vi "RES_HPSetup.vi"(8 "error in (no error)":errorcluster, 9 "Data Cluster In":T3 {"GUI Data Cluster"."SBR" format="%08b"}, 10 "Config Cluster In":T1={"General"={"Config.ini"=path "", "Default Logging Path"=path ""}, "Hardware"={"Measure Rate (1/s)"=0, "HP DMM VISA"="", "LS 335 VISA"="", "HP DM"={"Range"=enum."Autorange", "Autozero"=FALSE, "Display"=enum."3 1/2 Digit", "Blank LCD"=FALSE}}, "Operation"={"Operation Mode"=enum."Logging", "Status"="", "NewLog?"=FALSE, "OvenWarn"=FALSE}}) -> (0 "error out":errorcluster, 1 "Data Cluster Out":T3 {"GUI Data Cluster"."SBR" format="%08b"}, 2 "Config Cluster Out":T1={"General"={"Config.ini"=path "", "Default Logging Path"=path ""}, "Hardware"={"Measure Rate (1/s)"=0, "HP DMM VISA"="", "LS 335 VISA"="", "HP DM"={"Range"=enum."Autorange", "Autozero"=FALSE, "Display"=enum."3 1/2 Digit", "Blank LCD"=FALSE}}, "Operation"={"Operation Mode"=enum."Idle-Off", "Status"="", "NewLog?"=FALSE, "OvenWarn"=FALSE}})   [LabVIEW 2021]
uses:
  Config_Cluster.ctl
  Mode_Enum.ctl
  Data_Cluster.ctl
  Measurement_Cluster.ctl
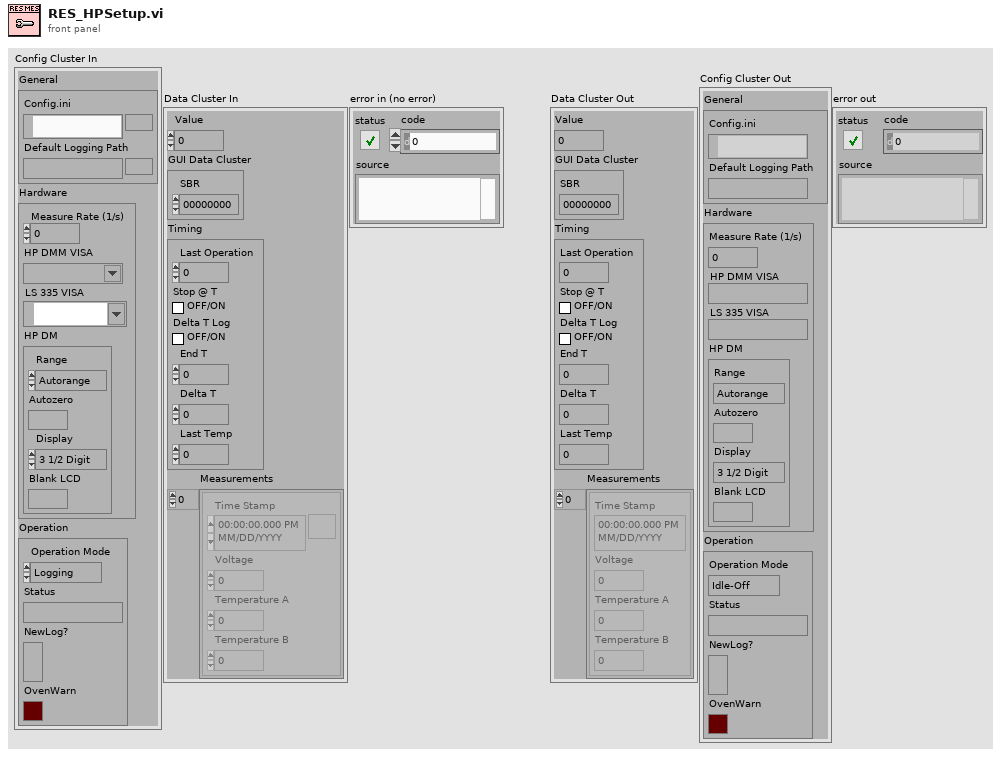
[diagram p1: front panel]
types:
  T1 = typedef "Config_Cluster.ctl" = cluster{"General":cluster{"Config.ini":path, "Default Logging Path":path}, "Hardware":cluster{"Measure Rate (1/s)":i32, "HP DMM VISA":refnum<visa-resource-name>, "LS 335 VISA":refnum<visa-resource-name>, "HP DM":cluster{"Range":enum16{"Autorange", "30mV", "300mV", "3V", "30V"}, "Autozero":bool, "Display":enum16{"3 1/2 Digit", "4 1/2 Digit", "5 1/2 Digit"}, "Blank LCD":bool}}, "Operation":cluster{"Operation Mode":T2, "Status":string, "NewLog?":bool, "OvenWarn":bool}}
  T2 = typedef "Mode_Enum.ctl" = enum16{"OvenNRDY", "Logging", "Idle-Off", "Idle"}
  T3 = typedef "Data_Cluster.ctl" = cluster{"Value":dbl, "GUI Data Cluster":cluster{"SBR":u16}, "Timing":cluster{"Last Operation":dbl, "Stop @ T":bool, "Delta T Log":bool, "End T":dbl, "Delta T":dbl, "Last Temp":dbl}, "Measurements":T4[]}
  T4 = typedef "Measurement_Cluster.ctl" = cluster{"Time Stamp":timestamp, "Voltage":dbl, "Temperature A":dbl, "Temperature B":dbl}
  T5 = cluster{"Range":enum16{"Autorange", "30mV", "300mV", "3V", "30V"}, "Autozero":bool, "Display":enum16{"3 1/2 Digit", "4 1/2 Digit", "5 1/2 Digit"}, "Blank LCD":bool}
  T6 = enum16{"Autorange", "30mV", "300mV", "3V", "30V"}
  T7 = enum16{"3 1/2 Digit", "4 1/2 Digit", "5 1/2 Digit"}
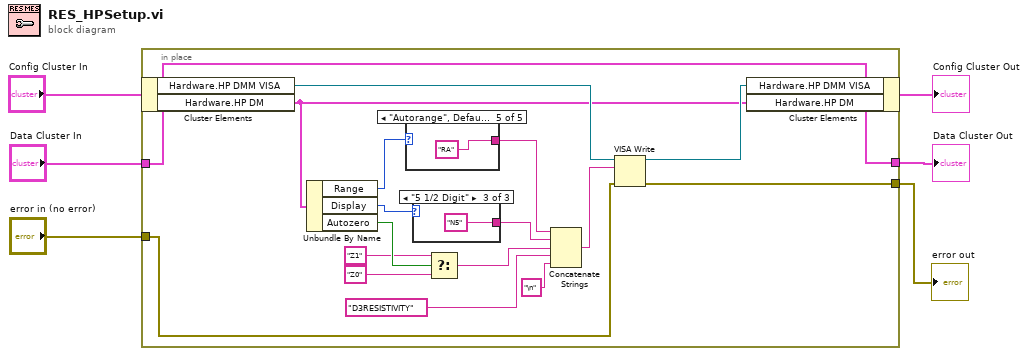
[diagram p0: block diagram]
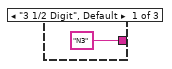
[diagram p2: hidden frame]
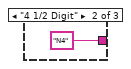
[diagram p3: hidden frame]
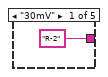
[diagram p4: hidden frame]
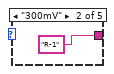
[diagram p5: hidden frame]
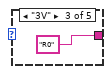
[diagram p6: hidden frame]
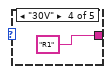
[diagram p7: hidden frame]
diagram:
  n1 = in-place {
    in-place-border: "Data Cluster In" -> [w10]
    in-place-border: "error in (no error)" -> [w13]
    in-place-border: [w10] -> w3
    in-place-border: [w9] -> w1
    n2 = in-place-cluster #1("Config Cluster In") -> ("Hardware.HP DMM VISA"=w15:refnum<visa-resource-name>, "Hardware.HP DM"=w11:T5)
    n3 = Unbundle By Name(w11) -> ("Range"=w23:T6, "Display"=w19:T7, "Autozero"=w22:bool)
    n4 = case shown="\"Autorange\", Default" w23 {
      tunnel: ["R-2" "R-1" "R0" "R1" "RA"] -> w18
      frame "30mV" {
      }
      frame "300mV" {
      }
      frame "3V" {
      }
      frame "30V" {
      }
      frame "Autorange", Default {
      }
    }
    n5 = case shown="\"5 1/2 Digit\"" w19 {
      tunnel: ["N3" "N4" "N5"] -> w17
      frame "3 1/2 Digit", Default {
      }
      frame "4 1/2 Digit" {
      }
      frame "5 1/2 Digit" {
      }
    }
    n6 = Select(t="Z1", s=w22, f="Z0") -> (s? t:f=w16:string)
    n7 = Concatenate Strings(w18, w17, w16, "D3RESISTIVITY", "\n" ("string")) -> (w14:string)
    n8 = VISA Write(VISA resource name=w15, write buffer=w14, error in (no error)=w13) -> (VISA resource name out=w12:refnum<visa-resource-name>, error out=w9:errorcluster)  [unwired: 1 out]
    n9 = in-place-cluster #1("Hardware.HP DMM VISA"=w12, "Hardware.HP DM"=w11) -> (→"Config Cluster Out":T1)
  }
  "Data Cluster Out" <- w3
  "error out" <- w1
